vi "task1_cosine_rule.vi"() -> ()   [LabVIEW 2020]
panel:
  in  "stop":bool
  out "angle_alpha_degree":dbl
  in  "c":dbl
  in  "b":dbl
  in  "a":dbl
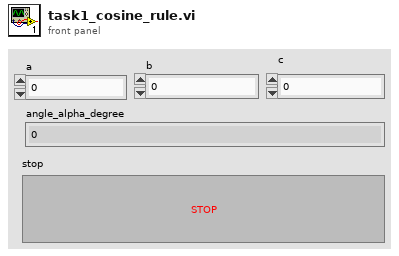
[diagram p1: front panel]
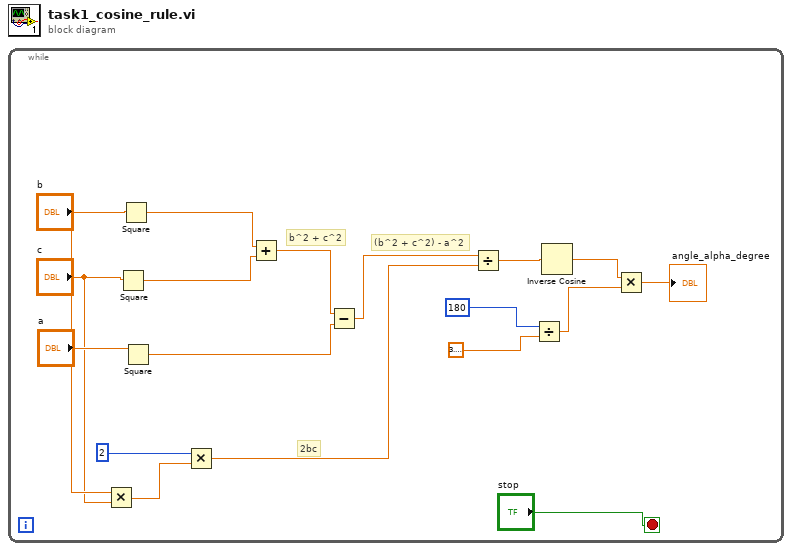
[diagram p0: block diagram]
diagram:
  n1 = while {
    stop <- "stop" stop-if-true
    # "(b^2 + c^2) - a^2"
    # "2bc"
    # "b^2 + c^2"
    n2 = Multiply(x="b", y="c") -> (x*y=w9:dbl)
    n3 = Square(x="c") -> (x^2=w15:dbl)
    n4 = Square(x="b") -> (x^2=w16:dbl)
    n5 = Square(x="a") -> (x^2=w13:dbl)
    n6 = Multiply(x=2, y=w9) -> (x*y=w8:dbl)
    n7 = Add(x=w16, y=w15) -> (x+y=w14:dbl)
    n8 = Subtract(x=w14, y=w13) -> (x-y=w7:dbl)
    n9 = Divide(x=w7, y=w8) -> (x/y=w6:dbl)
    n10 = Divide(x=180, y=3.141592653589793) -> (x/y=w2:dbl)
    n11 = Inverse Cosine(1:w6) -> (0:w3:dbl)
    n12 = Multiply(x=w3, y=w2) -> (x*y=→"angle_alpha_degree":dbl)
  }
